vi "Implement IIR Cascade Filter for N Chan (CDB).vi"(7 "reset filter states":bool[](array[boolean]), 8 "error in (no error)":errorcluster, 10 "IIR Filter Cluster":T1 {"Forward Coefficients" format="%0.4f"; "Reverse Coefficients" format="%0.4f"}, 11 "arrWaveforms":waveform(cdb)[](array[waveform])) -> (0 "error out":errorcluster, 3 "arrFilteredWaveforms":waveform(cdb)[](array[waveform]))   [LabVIEW 2020, in "NI_MAPro.lvlib"]
uses:
  NI_MAPro.lvlib
  NI_MABase.lvlib
  NI_AALBase.lvlib
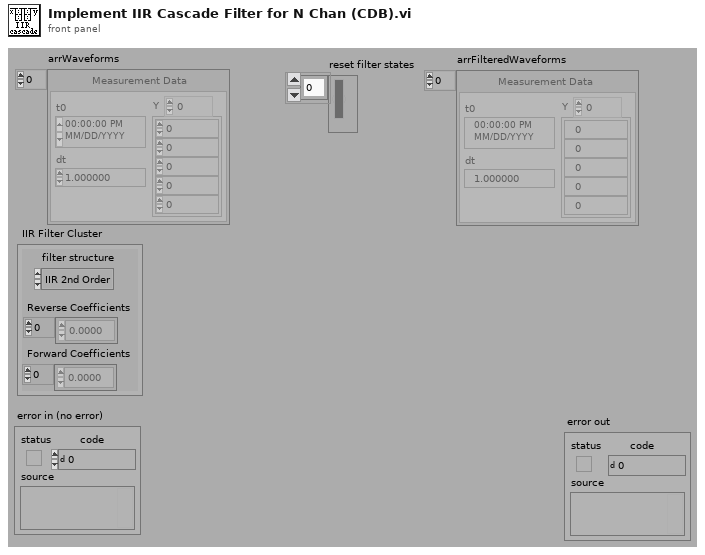
[diagram p1: front panel]
types:
  T1 = cluster{"filter structure":enum32{"IIR 2nd Order", "IIR 4th Order"}, "Reverse Coefficients":dbl[], "Forward Coefficients":dbl[]}
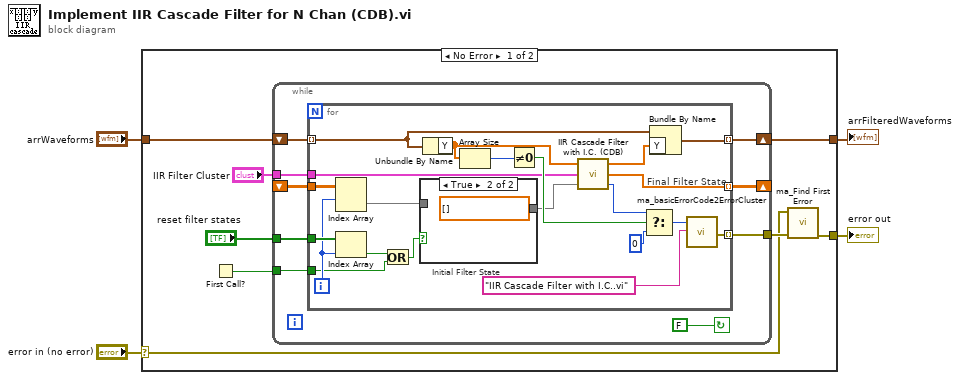
[diagram p0: block diagram]
diagram:
  n1 = case shown="No Error" "error in (no error)" {
    selector: "error in (no error)" -> [w10 w46]
    tunnel: [w11 w46] -> w3
    tunnel: "arrWaveforms" -> [w9 w45]
    tunnel: [w8 w45] -> w1
    frame No Error {
      n2 = First Call?() -> (First Call?: T/F=w6:bool)
      n3 = while {
        tunnel: "reset filter states" -> [w14]
        tunnel: [w15] -> w12
        tunnel: "IIR Filter Cluster" -> [w17]
        shift-left: w9 -> [w19]
        shift-right: [w18] -> w8
        shift-left: _ -> [w21]
        shift-right: [w20] -> _
        tunnel: w6 -> [w13]
        stop <- FALSE continue-if-true
        n4 = for {
          tunnel: w21 -> [w41]
          tunnel: [w36] -> w20 mode=indexing
          tunnel: w19 -> [w37] mode=indexing
          tunnel: [w40] -> w18 mode=indexing
          tunnel: w17 -> [w39]
          tunnel: [w31] -> w15 mode=indexing
          tunnel: w14 -> [w33]
          tunnel: w13 -> [w24]
          i -> [w32]
          # "Final Filter State"
          # "Initial Filter State"
          n5 = Index Array(array=w41, index (row)=w32) -> (element=w35:cdb[])  [unwired: 1 in]
          n6 = Index Array(array=w33, index=w32) -> (element=w23:bool)
          n7 = Or(x=w23, y=w24) -> (x .or. y?=w22:bool)
          n8 = case shown="True" w22 {
            tunnel: w35 -> [w43 _]
            tunnel: [w43 cdb[] [] ("Initial Filter State")] -> w34
            frame False {
            }
            frame True {
            }
          }
          n9 = Unbundle By Name(w37) -> ("Y"=w25:cdb[])
          n10 = Array Size(array=w25) -> (size(s)=w26:i32)
          n11 = Not Equal To 0?(x=w26) -> (x != 0?=w42:bool)
          n12 = call "IIR Cascade Filter with I.C. (CDB).vi"("Initial Filter State"=w34, "IIR Filter Cluster"=w39, "X"=w25) -> ("error"=w28:i32, "Final Filter State"=w36:cdb[], "Filtered X"=w38:cdb[])
          n13 = Select(t=w28, s=w42, f=0) -> (s? t:f=w27:i32)
          n14 = Bundle By Name(cluster=w37, "Y"=w38) -> (w40:waveform(cdb))
          n15 = call "ma_basicErrorCode2ErrorCluster.vi"("subVI name"="IIR Cascade Filter with I.C..vi", "Error Code"=w27) -> ("error out"=w31:errorcluster)  [unwired: 1 in]
        }
      }
      n16 = call "ma_Find First Error.vi"("error array in"=w12, "error in 1 (no error)"=w10) -> ("error out"=w11:errorcluster)  [unwired: 5 in]
    }
    frame Error {
    }
  }
  "error out" <- w3
  "arrFilteredWaveforms" <- w1
